vi "Sensor_Interface_Thread.vi"(8 "error in (no error)":errorcluster) -> (0 "error out":errorcluster)   [LabVIEW 2020]
doc: "Sensor Interface Thread"
uses:
  controls/FGV_To_Do.ctl
  controls/Share_Data.ctl
  controls/Configuration_Database.ctl
  controls/Event_User.ctl
  Controls/Sensor_Interface_Local_Variable.ctl
  Timer/Timer.lvclass
  SubVIs/Message Queue/Enqueue Message (Single).vi
  <vilib>/Utility/error.llb/Error Cluster From Error Code.vi
  <vilib>/ErrorRing/Error Ring.xnode
  SubVIs/User Event - Stop/User Event - Stop.lvlib
  SubVIs/Message Queue/Message Queue.lvlib
panel:
  in  "Elevator Position":u8(slide)=1 min=1 max=4 step=1 scale=1.0..4.0
  # "[Covers: UI1]"
  # "[Covers: UI4]"
  # "[Covers: UI4A]"
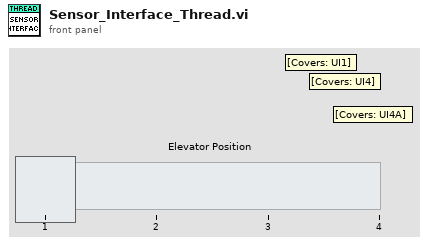
[diagram p1: front panel]
types:
  T1 = typedef "FGV_To_Do.ctl" = enum16{"1 - Initialize_Events", "2 - Read_Database", "3 - Initialize QMH", "Save_Database", "Read", "4 - Close_Events", "5 - Close_QMH"}
  T2 = typedef "All_Communication_Data.ctl" = cluster{"ConfigurationDatabase":T3, "QMH":T4, "User Event":T5}
  T3 = typedef "Configuration_Database.ctl" = cluster{"DoorOpen":u8, "DoorClose":u8, "TravelTime":u8, "InactivityTime":u8}
  T4 = typedef "Message Queue.lvlib/All Message Queues.ctl" = cluster{"UserConsole":refnum<queue>, "DisplayConsole":refnum<queue>, "SensorInterface":refnum<queue>}
  T5 = typedef "Event_User.ctl" = cluster{"User Event - Stop":refnum<user-event>, "User Event - Error":refnum<user-event>}
  T6 = typedef "Sensor_Interface_Local_Variable.ctl" = cluster{"Share_data":T7, "Elevator Position":refnum<vi>}
  T7 = typedef "Share_Data.ctl" = cluster{"ConfigurationDatabase":T3, "User Event":T5}
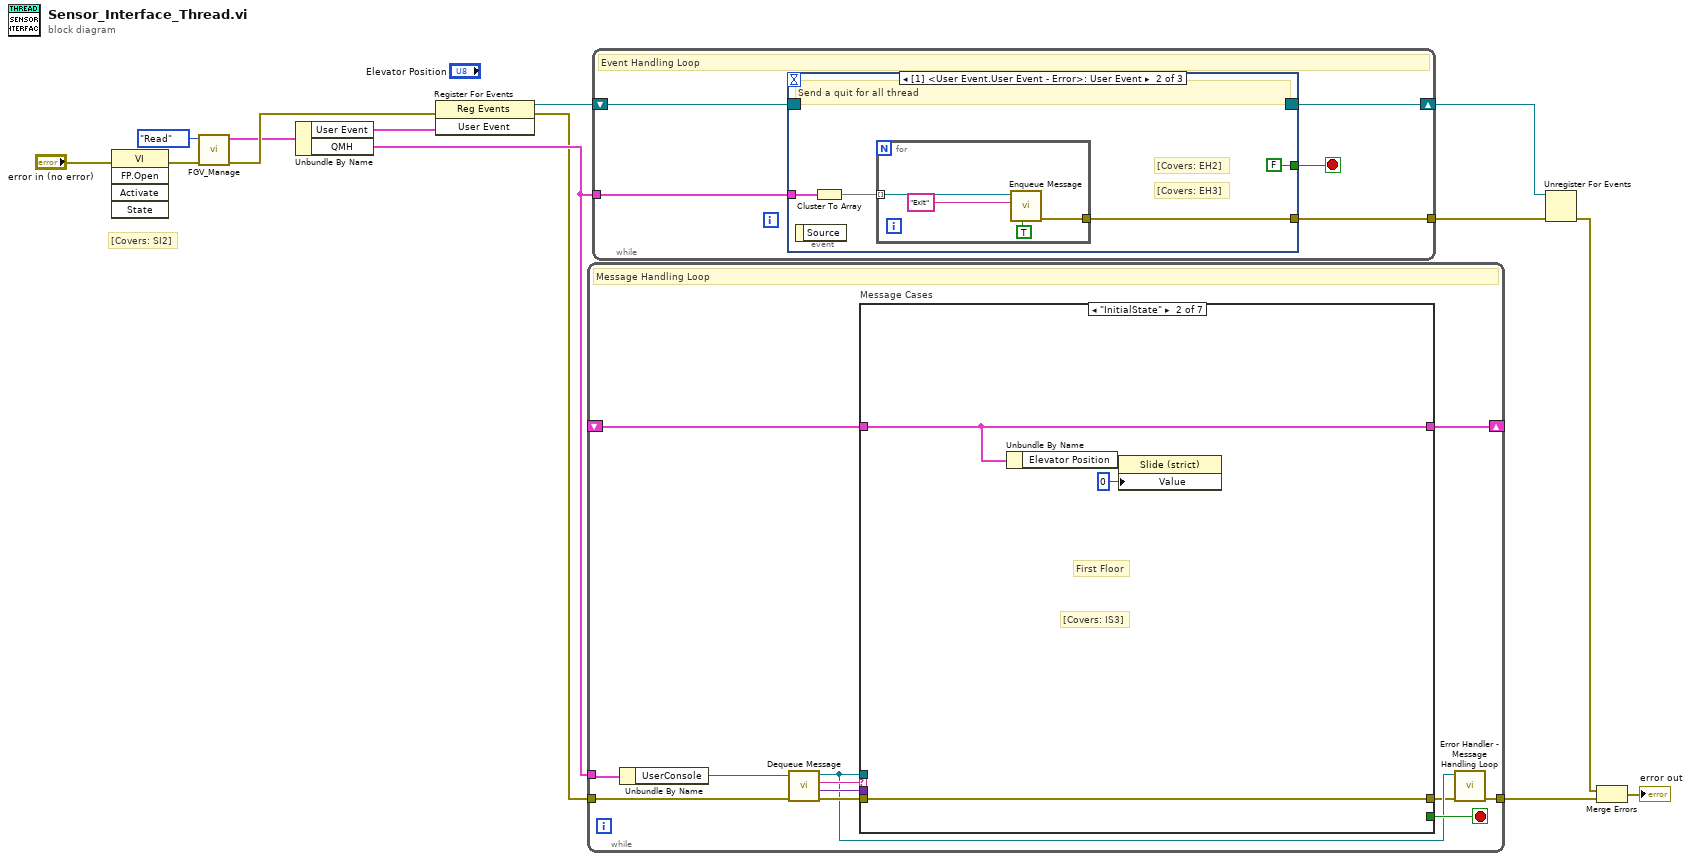
[diagram p0: block diagram]
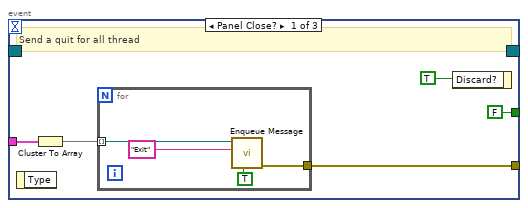
[diagram p2: hidden frame]
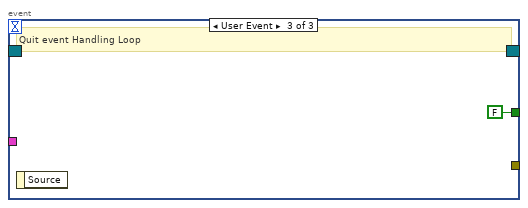
[diagram p3: hidden frame]
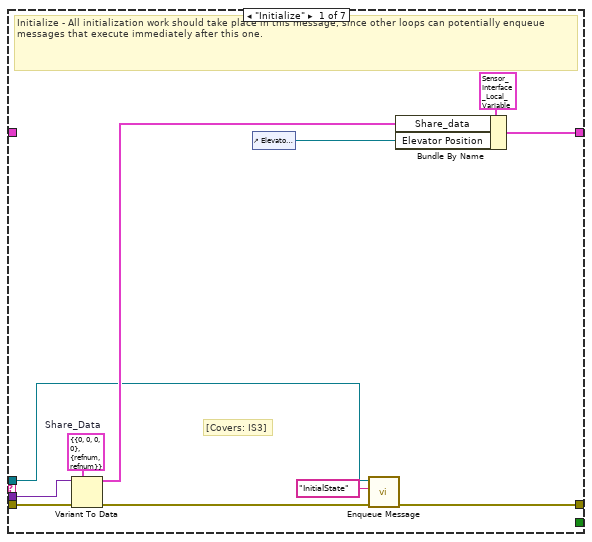
[diagram p4: hidden frame]
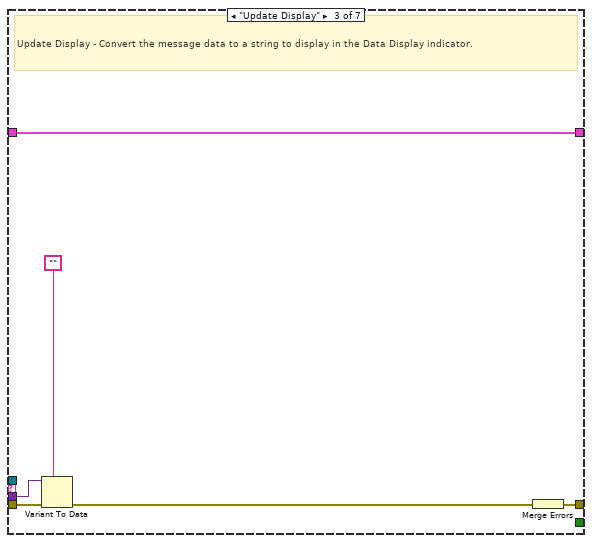
[diagram p5: hidden frame]
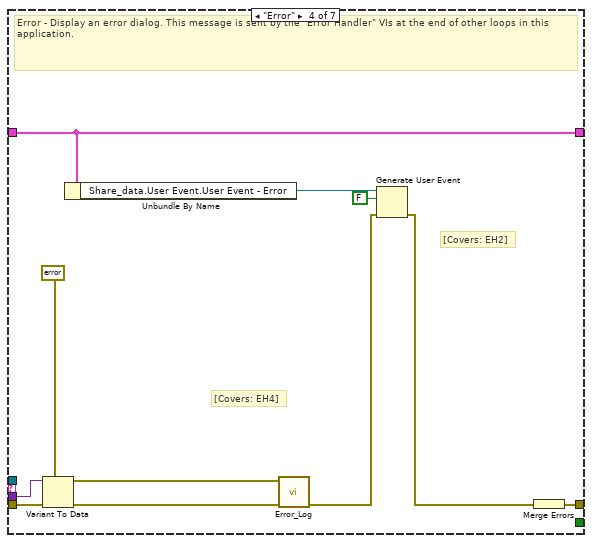
[diagram p6: hidden frame]
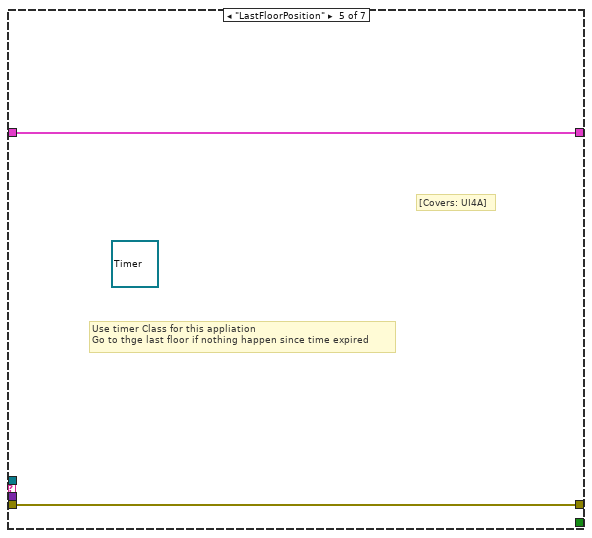
[diagram p7: hidden frame]
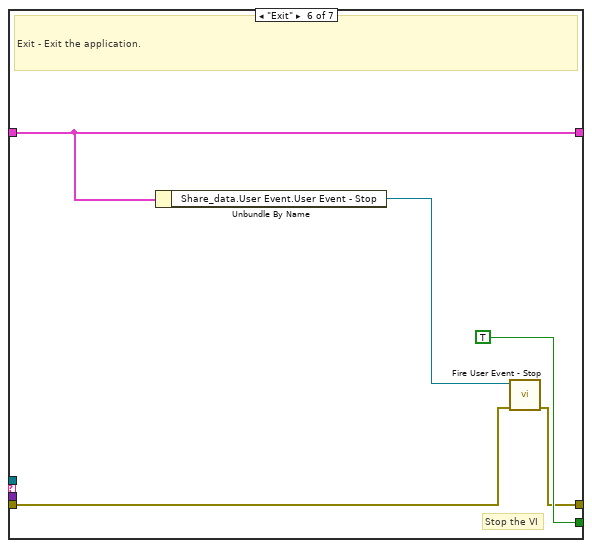
[diagram p8: hidden frame]
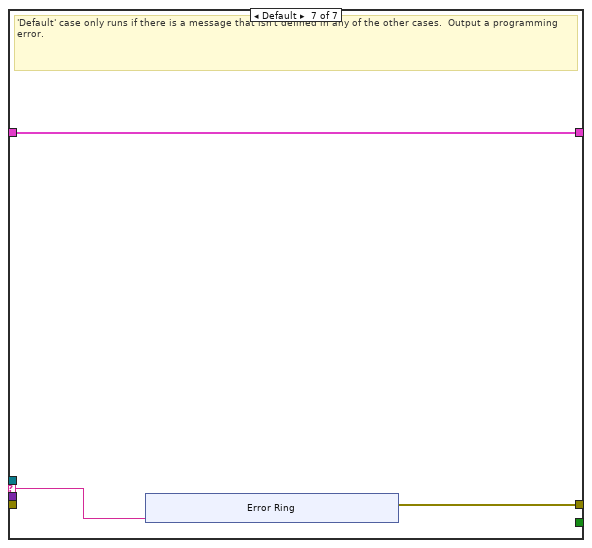
[diagram p9: hidden frame]
diagram:
  # "[Covers: SI2]"
  n1 = invoke class="VI" method="FP.Open"(error in="error in (no error)") -> (error out=w1:errorcluster)  [unwired: 4 in, 4 out]
  n2 = call "FGV_Manage.vi"("error in (no error)"=w1, "To do"=FGV_To_Do."Read") -> ("error out"=w11:errorcluster, "All_Communication OUT"=w9:T2)  [unwired: 8 in]
  n3 = Unbundle By Name(w9) -> ("User Event"=w10:T5, "QMH"=w13:T4)
  n4 = register-events(error in=w11, w10) -> (reference out=w7:refnum<event-registration>, error out=w12:errorcluster)  [unwired: 1 in]
  n5 = while {
    tunnel: w13 -> [w16]
    shift-right: [w25] -> _
    shift-left: _ -> [w26]
    tunnel: w12 -> [w23]
    tunnel: [w18] -> w3
    stop <- w24 stop-if-true
    # "Message Handling Loop"
    n6 = Unbundle By Name(w16) -> ("UserConsole"=w15:refnum<queue>)
    n7 = call "Dequeue Message.vi"("error in (no error)"=w23, "Message Queue"=w15) -> ("error out"=w22:errorcluster, "Message Data"=w20:variant, "Message"=w21:string, "dup Message Queue"=w19:refnum<queue>)  [unwired: 6 in]
    n8 = case "Message Cases" shown="\"InitialState\"" w21 {
      selector: w21 -> [_ _ _ _ _ _ w66]
      tunnel: w19 -> [w28 _ _ _ _ _ _]
      tunnel: w22 -> [w36 w41 w45 w58 w60 w62 _]
      tunnel: [w29 w41 w46 w55 w60 w61 w67] -> w17
      tunnel: w26 -> [_ w40 w47 w54 w59 w64 w68]
      tunnel: [w33 w40 w47 w54 w59 w64 w68] -> w25
      tunnel: [_ _ _ _ _ TRUE _] -> w24
      tunnel: w20 -> [w35 _ w44 w57 _ _ _]
      frame "Initialize" {
        w37 = T7 {"ConfigurationDatabase"={"DoorOpen"=0, "DoorClose"=0, "TravelTime"=0, "InactivityTime"=0}, "User Event"={"User Event - Stop"=refnum, "User Event - Error"=refnum}}  # Share_Data
        # "[Covers: IS3]"
        # "Initialize - All initialization work should take place in this message, since other loops can potentially enqueue messages that execute immediately after this one."
        n9 = Variant To Data(error in=w36, type=w37, Variant=w35) -> (data=w34:T7, error out=w30:errorcluster)
        n10 = control-ref of="Elevator Position"() -> (w31:refnum<vi>)
        n11 = call-poly "Enqueue Message.vi"("error in (no error)"=w30, "Message"="InitialState", "Message Queue"=w28) -> ("error out"=w29:errorcluster)  [unwired: 7 in, 1 out]
        n12 = Bundle By Name(cluster=T6 {"Share_data"={"ConfigurationDatabase"={"DoorOpen"=0, "DoorClose"=0, "TravelTime"=0, "InactivityTime"=0}, "User Event"={"User Event - Stop"=refnum, "User Event - Error"=refnum}}, "Elevator Position"=refnum} ("Local Variable"), "Share_data"=w34, "Elevator Position"=w31) -> (w33:T6)
      }
      frame "InitialState" {
        # "[Covers: IS3]"
        # "First Floor"
        n13 = Unbundle By Name(w40) -> ("Elevator Position"=w39:refnum<vi>)
        n14 = property class="Slide (strict)"(reference=w39, "Value"=u8 0) -> ()  [unwired: 1 in, 2 out]
      }
      frame "Update Display" {
        # "Update Display - Convert the message data to a string to display in the Data Display indicator."
        n15 = Variant To Data(error in=w45, type="", Variant=w44) -> (error out=w42:errorcluster)  [unwired: 1 out]
        n16 = Merge Errors(w42) -> (w46:errorcluster)
      }
      frame "Error" {
        # "[Covers: EH4]"
        # "[Covers: EH2]"
        # "Error - Display an error dialog. This message is sent by the \"Error Handler\" VIs at the end of other loops in this application."
        n17 = Variant To Data(error in=w58, type=errorcluster {"status"=FALSE, "code"=0, "source"=""} ("error constant"), Variant=w57) -> (data=w48:errorcluster, error out=w50:errorcluster)
        n18 = Unbundle By Name(w54) -> ("Share_data.User Event.User Event - Error"=w53:refnum<user-event>)
        n19 = call "Error_Log.vi"("error in"=w50, "Error report"=w48) -> ("error out"=w49:errorcluster)  [unwired: 9 in]
        n20 = Generate User Event(user event=w53, event data cluster=FALSE ("event data"), error in=w49) -> (error out=w51:errorcluster)  [unwired: 1 in, 1 out]
        n21 = Merge Errors(w51) -> (w55:errorcluster)
      }
      frame "LastFloorPosition" {
        (unwired) refnum<class "Timer.lvclass"> refnum ("Timer.lvclass")
        # "Use timer Class for this appliation\nGo to thge last floor if nothing happen since time expired"
        # "[Covers: UI4A]"
      }
      frame "Exit" {
        # "Stop the VI"
        # "Exit - Exit the application."
        n22 = Unbundle By Name(w64) -> ("Share_data.User Event.User Event - Stop"=w63:refnum<user-event>)
        n23 = call "Fire User Event - Stop.vi"("error in (no error)"=w62, "User Event - Stop"=w63) -> ("error out"=w61:errorcluster)  [unwired: 9 in]
      }
      frame Default {
        # "'Default' case only runs if there is a message that isn't defined in any of the other cases.  Output a programming error."
        n24 = xnode "Error Ring"("parameter 0"=w66) -> ("error out"=w67:errorcluster)
      }
    }
    n25 = call "Error Handler - Message Handling Loop.vi"("error in (no error)"=w17, "Message Queue"=w19) -> ("dup error in"=w18:errorcluster)  [unwired: 8 in, 1 out]
  }
  n26 = while {
    tunnel: w13 -> [w80]
    shift-right: [w78] -> w5
    shift-left: w7 -> [w79]
    tunnel: [w76] -> w6
    stop <- w77 stop-if-true
    # "Event Handling Loop"
    n27 = event shown="[1] <User Event.User Event - Error>: User Event" {
      selector: w79 -> [_ _ _]
      dyn-events: [_ _ _] -> w78
      timeout: _ -> [_ _ _]
      tunnel: [FALSE ("Discard?") FALSE ("Discard?") FALSE ("Discard?")] -> w77
      tunnel: w80 -> [w84 w93 _]
      tunnel: [w83 w92 _] -> w76
      event Panel Close? {
        # "Send a quit for all thread"
        n28 = event-data() -> ()  [unwired: 1 in, 1 out]
        n29 = Cluster To Array(cluster=w84) -> (array=w82:refnum<queue>[])
        n30 = for {
          tunnel: w82 -> [w89] mode=indexing
          tunnel: [w88] -> w83
          n31 = call-poly "Enqueue Message.vi"("Priority Message? (F)"=TRUE, "Message"="Exit", "Message Queue"=w89) -> ("error out"=w88:errorcluster)  [unwired: 7 in, 1 out]
        }
        n32 = event-data("Discard?"=TRUE) -> ()  [unwired: 1 in, 1 out]
      }
      event User Event {
        # "[Covers: EH3]"
        # "[Covers: EH2]"
        # "Send a quit for all thread"
        n33 = event-data() -> ()  [unwired: 1 in, 1 out]
        n34 = Cluster To Array(cluster=w93) -> (array=w91:refnum<queue>[])
        n35 = for {
          tunnel: w91 -> [w97] mode=indexing
          tunnel: [w96] -> w92
          n36 = call-poly "Enqueue Message.vi"("Priority Message? (F)"=TRUE, "Message"="Exit", "Message Queue"=w97) -> ("error out"=w96:errorcluster)  [unwired: 7 in, 1 out]
        }
      }
      event User Event {
        # "Quit event Handling Loop"
        n37 = event-data() -> ()  [unwired: 1 in, 1 out]
      }
    }
  }
  n38 = Unregister For Events(event registration refnum=w5, error in=w6) -> (error out=w4:errorcluster)
  n39 = Merge Errors(w4, w3) -> (→"error out":errorcluster)
